vi "Controll Inputs (SubVI).vi"(8 "error in (no error)":errorcluster, 10 "Manual":bool=TRUE, 11 "Refnum in":refnum<k1>) -> (0 "error out":errorcluster, 1 "Land/Take off":bool, 2 "Boolean":bool, 3 "Control cluster":T1)   [LabVIEW 2014]
uses:
  Global.vi
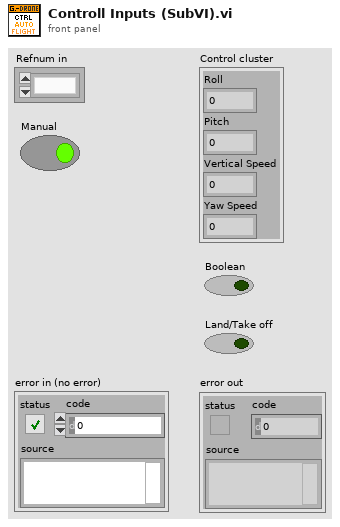
[diagram p1: front panel]
types:
  T1 = cluster{"Roll":dbl, "Pitch":dbl, "Vertical Speed":dbl, "Yaw Speed":dbl}
  T2 = cluster{"Hover":bool, "Land/Take off":bool, "button 3":bool, "button 4":bool}
  T3 = typedef "Control cluster.ctl" = cluster{"Roll":sgl, "Pitch":sgl, "Vertical Speed":sgl, "Yaw Speed":sgl}
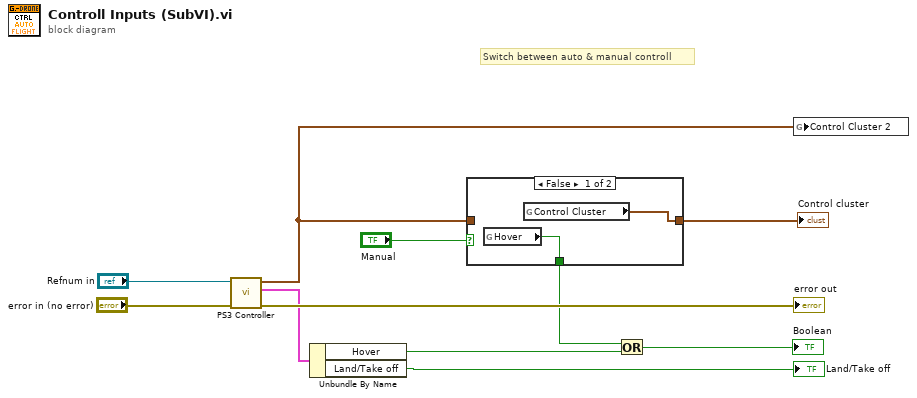
[diagram p0: block diagram]
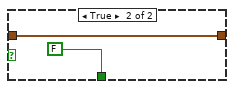
[diagram p2: hidden frame]
diagram:
  # "Switch between auto & manual controll"
  n1 = call "PS3 Controller.vi"("error in (no error)"="error in (no error)", "device ID"="Refnum in") -> ("error out"=→"error out":errorcluster, "Buttons control"=w4:T2, "Control cluster"=w8:T1)  [unwired: 7 in]
  n2 = Unbundle By Name(w4) -> ("Hover"=w3:bool, "Land/Take off"=→"Land/Take off":bool)
  n3 = case shown="False" "Manual" {
    tunnel: w8 -> [_ w14]
    tunnel: [w13 w14] -> w7
    tunnel: [w12 FALSE] -> w2
    frame False {
      n4 = global read "Global.vi" "Hover"() -> (w12:bool)
      n5 = global read "Global.vi" "Control Cluster"() -> (w13:T3)
    }
    frame True {
    }
  }
  "Control cluster" <- w7
  n6 = Or(x=w2, y=w3) -> (x .or. y?=→"Boolean":bool)
  n7 = global write "Global.vi" "Control Cluster 2"(w8) -> ()
